vi "True.vi"() -> ()   [LabVIEW 2016, in "test_AssertControlValue.lvlib"]
uses:
  test_AssertControlValue.lvlib
  main/apis/Setup/GetVI/GetVIByPath.vi
  main/apis/Stimulus/ValueSignal/ValueSignalByPathString.vi
  main/apis/Setup/GetVI/GetVI.lvlib
  <vilib>/addons/_JKI Toolkits/Caraya/classes/Test/Test.lvclass
  main/apis/Assert/AssertControlValue/AssertControlValue.lvlib
panel:
  out "error out":errorcluster
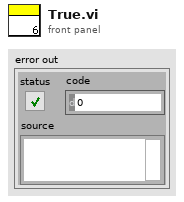
[diagram p1: front panel]
types:
  T1 = enum32{"Invalid", "Standard", "Closed", "Hidden", "Minimized", "Maximized"}
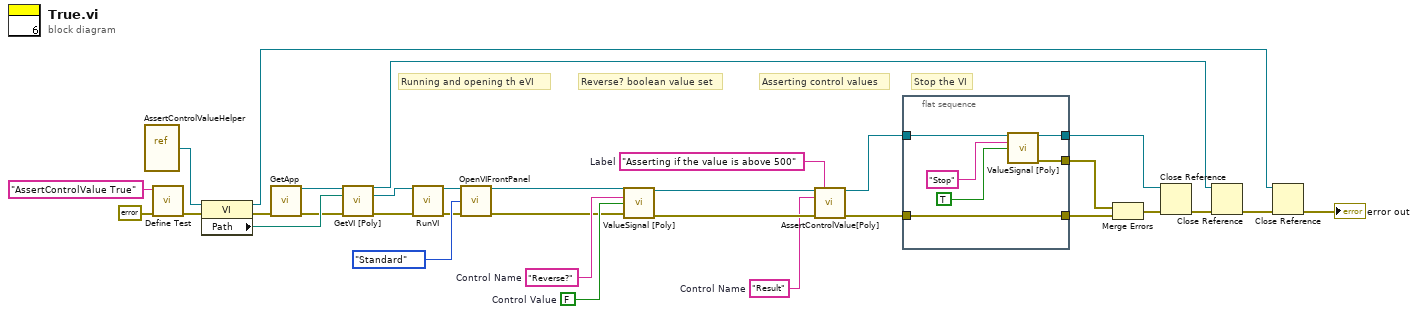
[diagram p0: block diagram]
diagram:
  w1 = "Asserting if the value is above 500"  # Label
  w18 = "Result"  # Control Name
  w27 = FALSE  # Control Value
  w28 = "Reverse?"  # Control Name
  # "Running and opening th eVI"
  # "Reverse? boolean value set"
  # "Asserting control values"
  # "Stop the VI"
  n1 = vi-ref "AssertControlValueHelper.vi"() -> (w22:refnum<vi>)
  n2 = call <vilib>:"Define Test.vi"("error in (no error)"=errorcluster {"status"=FALSE, "code"=0, "source"=""}, "Label (VI Title)"="AssertControlValue True") -> ("error out"=w23:errorcluster)  [unwired: 9 in]
  n3 = property on="Property Node" class="VI"(reference=w22, error in=w23) -> (reference out=w2:refnum<vi>, error out=w31:errorcluster, "Path"=w30:path)
  n4 = call "GetApp.vi"("error in (no error)"=w31) -> ("Application Ref"=w32:refnum<vi>, "error out"=w29:errorcluster)  [unwired: 13 in]
  n5 = call-poly "GetVI [Poly].vi"("Application Ref in"=w32, "VI Path"=w30, "error in (no error)"=w29) -> ("Application Ref out"=w3:refnum<vi>, "VI Reference"=w26:refnum<vi>, "error out"=w25:errorcluster)  [unwired: 10 in]
  n6 = call "RunVI.vi"("VI Reference In"=w26, "error in"=w25) -> ("VI Reference Out"=w6:refnum<vi>, "error out"=w7:errorcluster)  [unwired: 12 in]
  n7 = call "OpenVIFrontPanel.vi"("VI Reference In"=w6, "State(Standard)"=T1."Standard", "error in"=w7) -> ("VI Reference Out"=w10:refnum<vi>, "error out"=w9:errorcluster)  [unwired: 11 in]
  n8 = call-poly "ValueSignal [Poly].vi"("VI Reference In"=w10, "Control Name"=w28, "Value (Signaling)"=w27, "error in"=w9) -> ("VI Reference Out"=w19:refnum<vi>, "error out"=w20:errorcluster)  [unwired: 10 in]
  n9 = call-poly "AssertControlValue[Poly].vi"("VI Reference In"=w19, "Label"=w1, "Control Name"=w18, "Error In"=w20) -> ("VI Reference Out"=w17:refnum<vi>, "Error Out"=w16:errorcluster)  [unwired: 10 in]
  n10 = flat-sequence {
    tunnel: w17 -> [w36]
    tunnel: [w35] -> w15
    tunnel: w16 -> [w34]
    tunnel: [w34] -> w14
    tunnel: [w33] -> w11
    frame #0 {
      n11 = call-poly "ValueSignal [Poly].vi"("VI Reference In"=w36, "Control Name"="Stop" ("Class Name"), "Value (Signaling)"=TRUE) -> ("VI Reference Out"=w33:refnum<vi>, "error out"=w35:errorcluster)  [unwired: 11 in]
    }
  }
  n12 = Merge Errors(w15, w14) -> (w13:errorcluster)
  n13 = Close Reference(reference=w11, error in (no error)=w13) -> (error out=w12:errorcluster)
  n14 = Close Reference(reference=w3, error in (no error)=w12) -> (error out=w5:errorcluster)
  n15 = Close Reference(reference=w2, error in (no error)=w5) -> (error out=→"error out":errorcluster)
